vi "ReadTargetDoseNode.vi"(8 "Error In":errorcluster, 11 "Experiment Node In":refnum<k20>) -> (0 "Error Out":errorcluster, 2 "Target Dose (dpa)":dbl, 3 "Experiment Node Out":refnum<k20>)   [LabVIEW 2012]
uses:
  <vilib>/xml/NI_XML.lvlib
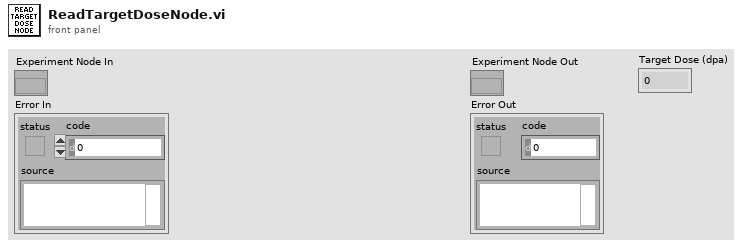
[diagram p1: front panel]
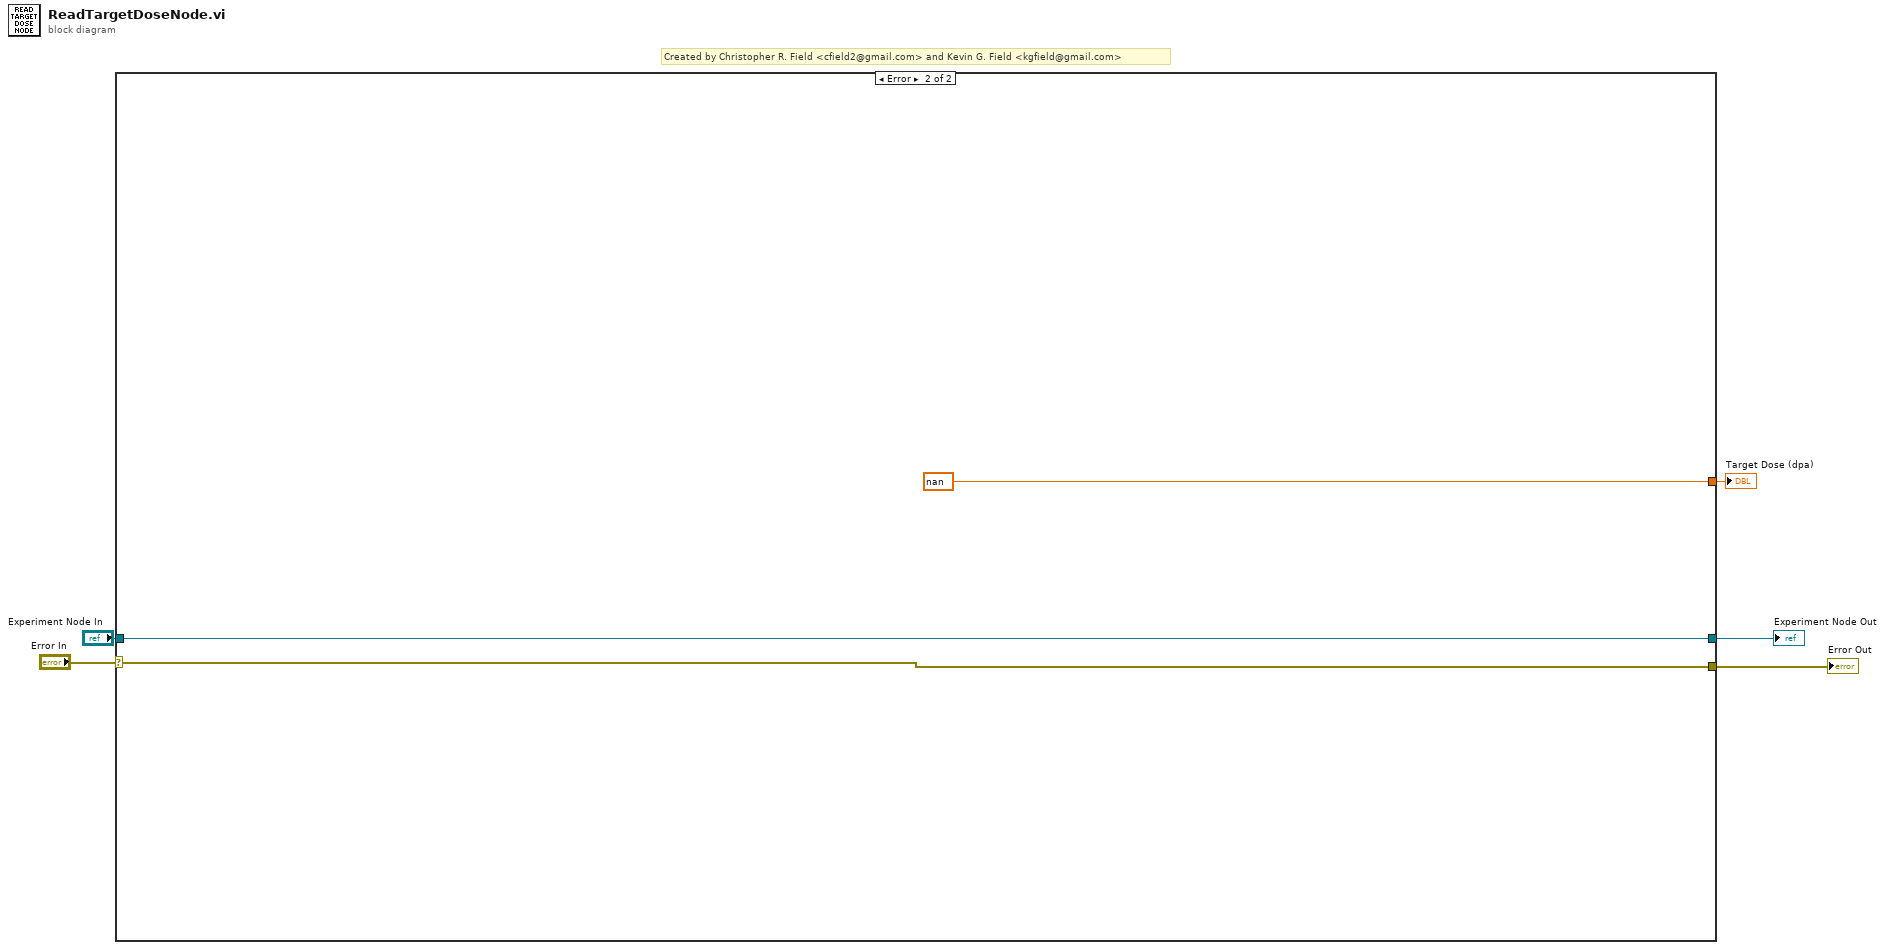
[diagram p0: block diagram]
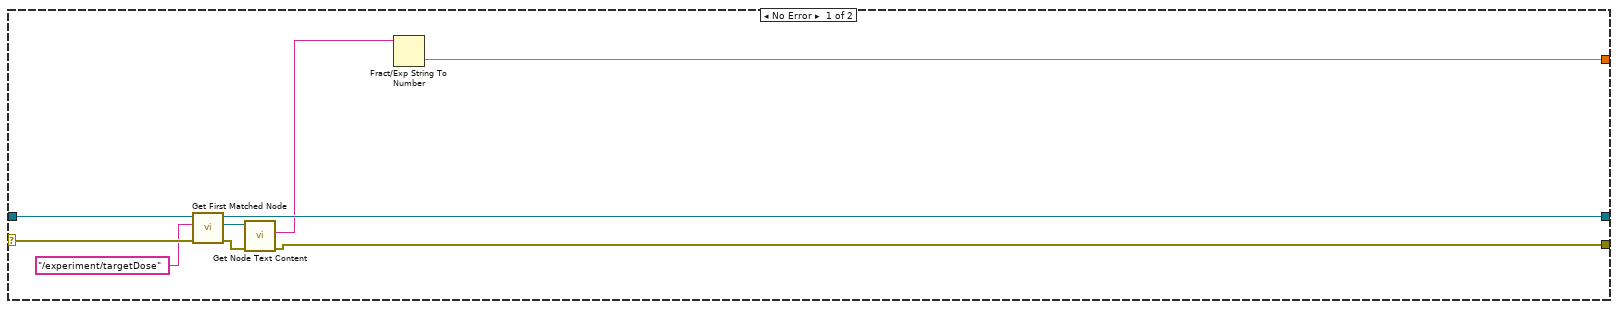
[diagram p2: hidden frame]
diagram:
  # "Created by Christopher R. Field <cfield2@gmail.com> and Kevin G. Field <kgfield@gmail.com>"
  n1 = case shown="Error" "Error In" {
    selector: "Error In" -> [w13 w16]
    tunnel: "Experiment Node In" -> [w14 w17]
    tunnel: [w9 w17] -> w3
    tunnel: [w8 w16] -> w2
    tunnel: [w6 nan] -> w1
    frame No Error {
      n2 = call <vilib>:"Get First Matched Node.vi"("error in (no error)"=w13, "XPath expression"="/experiment/targetDose", "node in"=w14) -> ("error out"=w10:errorcluster, "node result"=w11:refnum<k20>, "node out"=w9:refnum<k20>)  [unwired: 6 in]
      n3 = call <vilib>:"Get Node Text Content.vi"("error in (no error)"=w10, "node in"=w11) -> ("error out"=w8:errorcluster, "node text"=w7:string)  [unwired: 7 in, 1 out]
      n4 = Fract/Exp String To Number(string=w7) -> (number=w6:dbl)  [unwired: 3 in, 1 out]
    }
    frame Error {
    }
  }
  "Experiment Node Out" <- w3
  "Error Out" <- w2
  "Target Dose (dpa)" <- w1
